vi "3.1.1.1-VectorNav Read.vi"() -> (2 "Reply":string)   [LabVIEW 2010]
uses:
  3.1.1.1-VectorNav Parser.ctl
  <vilib>/userDefined/High Color/nirio_resource_hc.ctl
  <vilib>/rvi/interface/nirviOpenFPGA/nirviOpenFPGA.xnode
  FPGA Bitfiles/DaveBrain_FPGATarget_1.2.1.1-VectorNa_98C397BE.lvbitx
  1-Hindbrain/1.2-Where/1.2.1-VectorNav/1.2.1.1-VectorNav Read Write.vi
  <vilib>/rvi/ClientSDK/nirviWhatTheDeviceIsDoing.ctl
  <vilib>/rvi/interface/nirviMethod/nirviMethod.xnode
  <vilib>/rvi/interface/common/niFpgaNodeNameForErrorReporting.ctl
  <vilib>/rvi/errors/niLvFpgaWhatHappensToTopLevelVI.ctl
  <vilib>/rvi/interface/nirviCloseFPGA/nirviCloseFPGA.xnode
  <vilib>/FPGAPlugInAG/cRIO-9104/niLvFpga_Open_cRIO-9104.vi
  <vilib>/rvi/interface/common/dynamic/niFpgaDynamicAddResources.vi
  <vilib>/Utility/error.llb/Error Cluster From Error Code.vi
  <vilib>/rvi/errors/niLvFpgaAdjustHostInterfaceError.vi
  <vilib>/FPGAPlugInAG/Dynamic/niLvFpga_Close_Dynamic.vi
  NiFpgaLv.dll
panel:
  out "Data":string
  out "error IO":errorcluster
  out "Elements Remaining":u32
  out "Enum":T1
  out "Checksum":string
  out "String":string
  in  "stop":bool
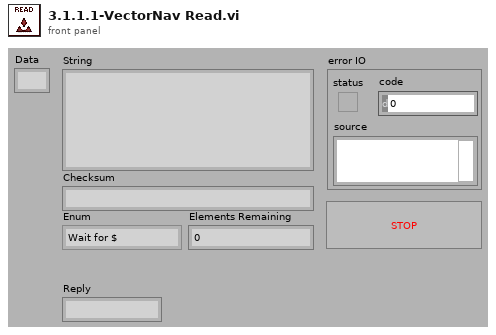
[diagram p1: front panel]
types:
  T1 = typedef "3.1.1.1-VectorNav Parser.ctl" = enum16{"Wait for $", "Read values", "Checksum", "Error", "Done"}
  T2 = typedef "niFpgaNodeNameForErrorReporting.ctl" = enum16{"Open FPGA VI Reference", "Read/Write Control", "Invoke Method: Abort", "Invoke Method: Acknowledge IRQ", "Invoke Method: Download", "Invoke Method: FIFO.Configure", "Invoke Method: FIFO.Read", "Invoke Method: FIFO.Start", "Invoke Method: FIFO.Stop", "Invoke Method: FIFO.Write", "Invoke Method: Reset", "Invoke Method: Run", "Invoke Method: Wait on IRQ", "Close FPGA VI Reference"}
  T3 = typedef "niLvFpgaWhatHappensToTopLevelVI.ctl" = enum16{"top level VI scripted behind XNode", "top level VI inlined behind XNode"}
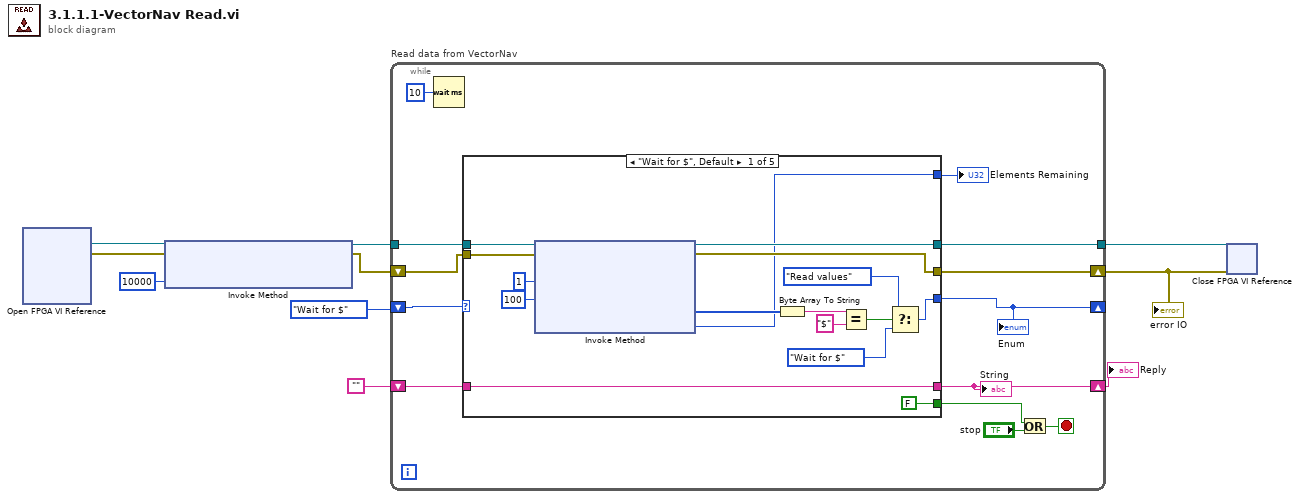
[diagram p0: block diagram]
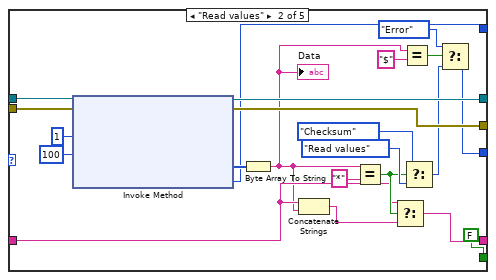
[diagram p2: hidden frame]
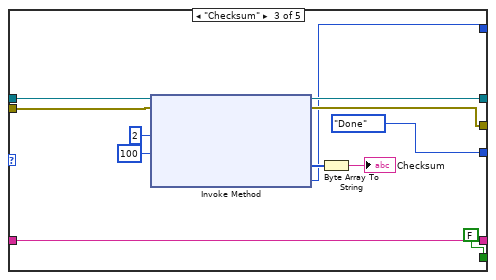
[diagram p3: hidden frame]
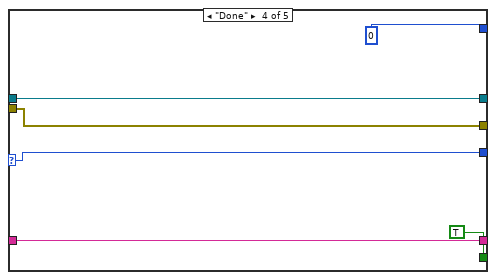
[diagram p4: hidden frame]
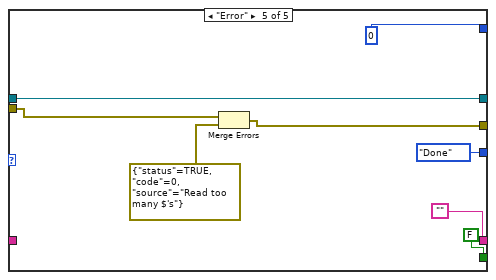
[diagram p5: hidden frame]
diagram:
  n1 = xnode "Open FPGA VI Reference"() -> ("FPGA VI Reference Out"=w1:refnum<k20>, "error out"=w10:errorcluster)  [unwired: 2 in]
  n2 = xnode "Invoke Method"("FPGA VI Reference In"=w1, "error in"=w10, "Depth"=u32 10000) -> ("FPGA VI Reference Out"=w8:refnum<k20>, "error out"=w7:errorcluster)
  n3 = while "Read data from VectorNav" {
    tunnel: w8 -> [w16]
    tunnel: [w14] -> w6
    shift-right: [w11] -> w2
    shift-left: "" -> [w18]
    shift-right: [w20] -> _
    shift-left: 3.1.1.1-VectorNav_Parser."Wait for $" ("Enum") -> [w19]
    shift-right: [w13] -> w5
    shift-left: w7 -> [w15]
    stop <- w21 stop-if-true
    n4 = Wait (ms)(milliseconds to wait=u32 10) -> ()  [unwired: 1 out]
    n5 = case shown="\"Wait for $\", Default" w19 {
      selector: w19 -> [_ _ _ w294 _]
      tunnel: [w31 w113 3.1.1.1-VectorNav_Parser."Done" ("Enum") w294 3.1.1.1-VectorNav_Parser."Done" ("Enum")] -> w20
      tunnel: w18 -> [w30 w126 w214 w298 _]
      tunnel: [w30 w125 w214 w298 ""] -> w11
      tunnel: [FALSE FALSE FALSE TRUE FALSE] -> w17
      tunnel: w16 -> [w28 w123 w212 w296 w304]
      tunnel: w15 -> [w27 w122 w211 w295 w306]
      tunnel: [w26 w121 w210 w296 w304] -> w14
      tunnel: [w25 w120 w209 w295 w305] -> w13
      tunnel: [w24 w119 w208 u32 0 ("Elements Remaining") u32 0 ("Elements Remaining")] -> w12
      frame "Wait for $", Default {
        n6 = xnode "Invoke Method"("FPGA VI Reference In"=w28, "error in"=w27, "Number of Elements"=u32 1, "Timeout (ms)"=100) -> ("FPGA VI Reference Out"=w26:refnum<k20>, "error out"=w25:errorcluster, "Data"=w39:u8[], "Elements Remaining"=w24:u32)
        n7 = Byte Array To String(unsigned byte array=w39) -> (string=w34:string)
        n8 = Equal?(x=w34, y="$") -> (x = y?=w35:bool)
        n9 = Select(t=3.1.1.1-VectorNav_Parser."Read values" ("Enum"), s=w35, f=3.1.1.1-VectorNav_Parser."Wait for $" ("Enum")) -> (s? t:f=w31:T1)
      }
      frame "Read values" {
        n10 = xnode "Invoke Method"("FPGA VI Reference In"=w123, "error in"=w122, "Number of Elements"=u32 1, "Timeout (ms)"=100) -> ("FPGA VI Reference Out"=w121:refnum<k20>, "error out"=w120:errorcluster, "Data"=w129:u8[], "Elements Remaining"=w119:u32)
        n11 = Byte Array To String(unsigned byte array=w129) -> (string=w117:string)
        "Data" <- w117
        n12 = Concatenate Strings(w126, w117) -> (w127:string)
        n13 = Equal?(x=w117, y="*") -> (x = y?=w128:bool)
        n14 = Select(t=w126, s=w128, f=w127) -> (s? t:f=w125:string)
        n15 = Equal?(x=w117, y="$") -> (x = y?=w116:bool)
        n16 = Select(t=3.1.1.1-VectorNav_Parser."Checksum" ("Enum"), s=w128, f=3.1.1.1-VectorNav_Parser."Read values" ("Enum")) -> (s? t:f=w114:T1)
        n17 = Select(t=3.1.1.1-VectorNav_Parser."Error" ("Enum"), s=w116, f=w114) -> (s? t:f=w113:T1)
      }
      frame "Checksum" {
        n18 = xnode "Invoke Method"("FPGA VI Reference In"=w212, "error in"=w211, "Number of Elements"=u32 2, "Timeout (ms)"=100) -> ("FPGA VI Reference Out"=w210:refnum<k20>, "error out"=w209:errorcluster, "Data"=w217:u8[], "Elements Remaining"=w208:u32)
        n19 = Byte Array To String(unsigned byte array=w217) -> (string=→"Checksum":string)
      }
      frame "Done" {
      }
      frame "Error" {
        n20 = Merge Errors(w306, errorcluster {"status"=TRUE, "code"=0, "source"="Read too many $'s"} ("error in")) -> (w305:errorcluster)
      }
    }
    "Enum" <- w20
    "Elements Remaining" <- w12
    "String" <- w11
    n21 = Or(x=w17, y="stop") -> (x .or. y?=w21:bool)
  }
  "error IO" <- w5
  "Reply" <- w2
  n22 = xnode "Close FPGA VI Reference"("FPGA VI Reference In"=w6, "error in"=w5) -> ()  [unwired: 1 out]
